vi "Select XNET Signals UI.vi"(8 "error in (no error)":errorcluster, 9 "XNET Cluster":refnum<k21>, 10 "XNET Database":refnum<k21>, 11 "Node Ptr":u64 format="%.0x") -> (0 "error out":errorcluster, 2 "Cancel Out":bool)   [LabVIEW 2019, in "Ghost Bus Addon System Explorer.lvlib"]
uses:
  Ghost Bus Addon System Explorer.lvlib
  <vilib>/Utility/cursorutil.llb/Set Cursor (Icon Pict).vi
panel:
  in  "Cancel":bool
  in  "Select":bool
  in  "Tree":string(tree)
  # "OUTPUTS"
  # "INPUTS"
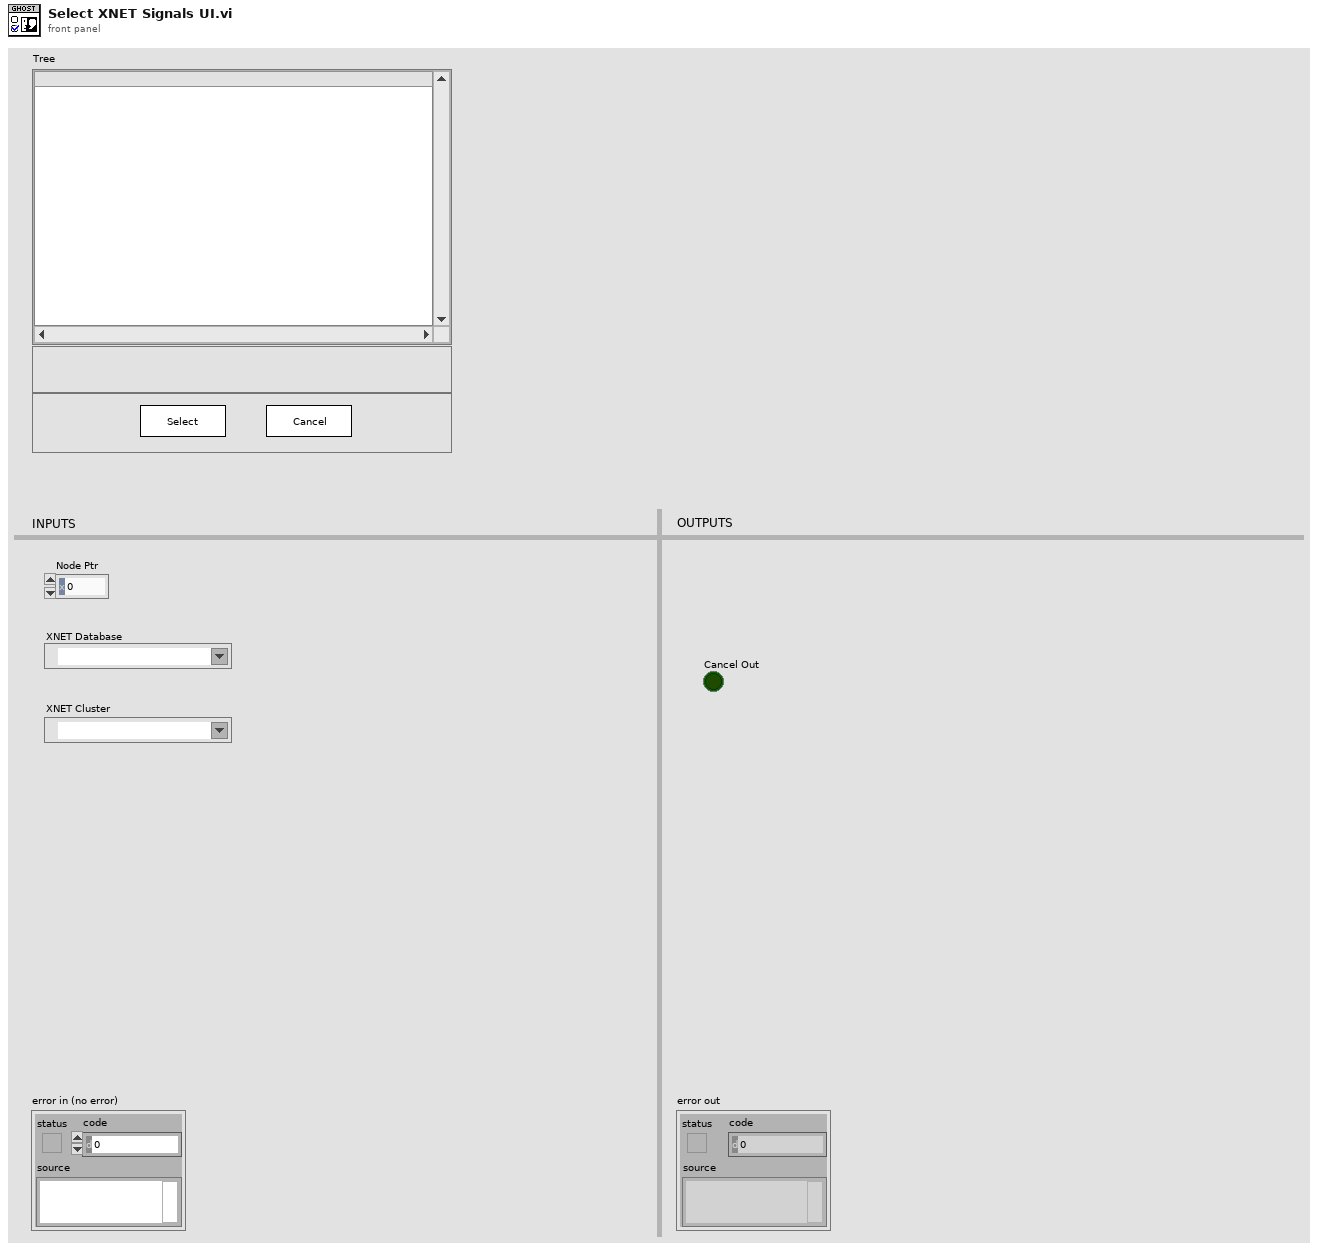
[diagram p1: front panel]
types:
  T1 = typedef "LVPoint32TypeDef.ctl" = cluster{"Horizontal":i32, "Vertical":i32}
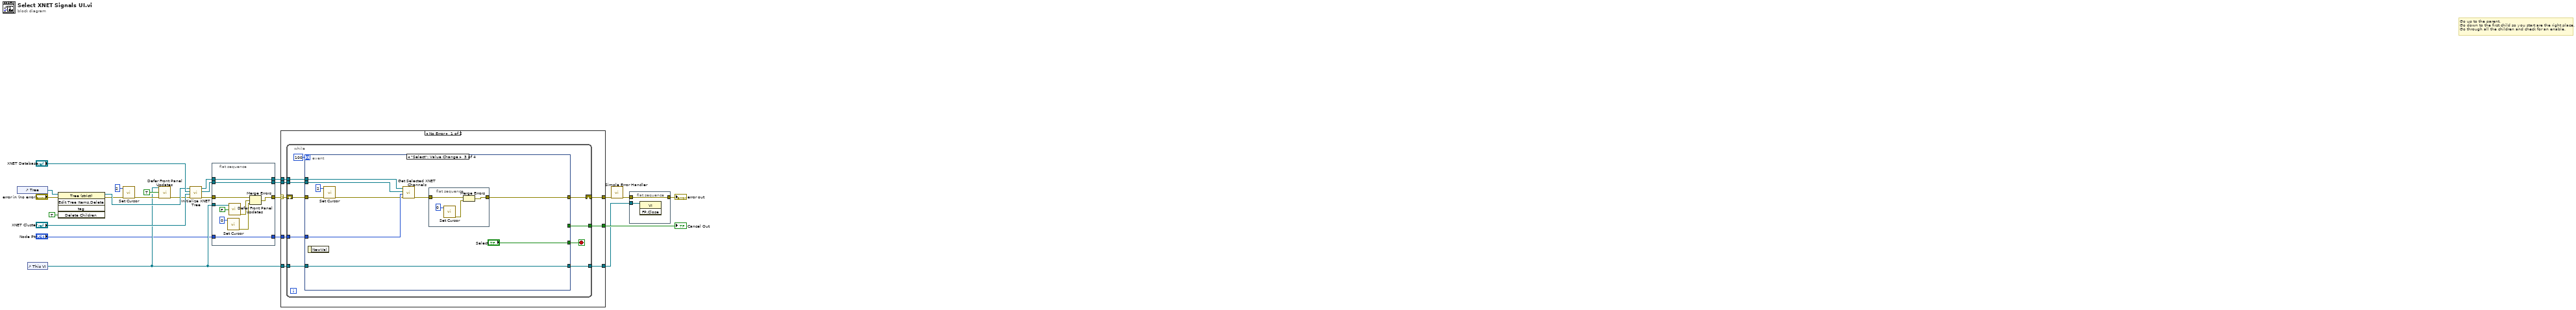
[diagram p0: block diagram]
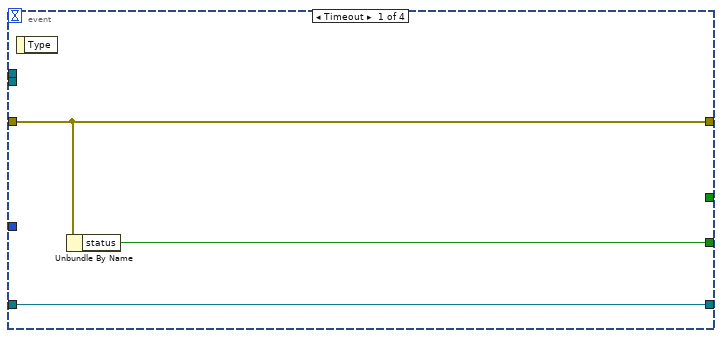
[diagram p2: hidden frame]
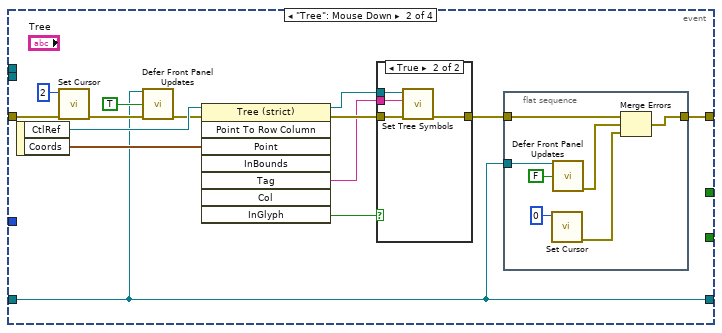
[diagram p3: hidden frame]
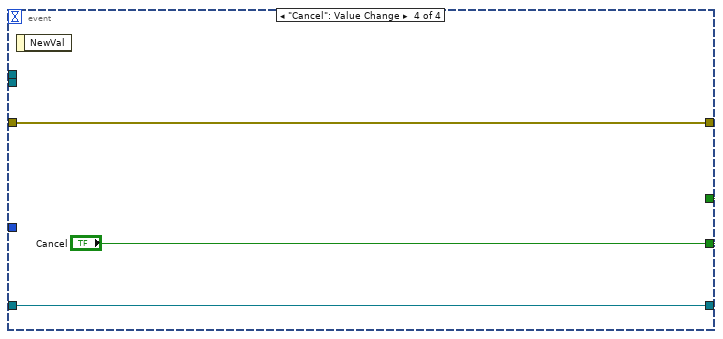
[diagram p5: hidden frame]
diagram:
  # "Go up to the parent.\nGo down to the first child so you start are the right place.\nGo through all the children and check for an enable."
  n1 = control-ref of="Tree"() -> (w13:refnum<vi>)
  n2 = control-ref of="This VI"() -> (w6:refnum<vi>)
  n3 = invoke on="Invoke Node" class="Tree (strict)" method="Edit Tree Items.Delete"(reference=w13, error in="error in (no error)", "Delete Children"=TRUE ("Delete Children?")) -> (reference out=w12:refnum<vi>, error out=w10:errorcluster)  [unwired: 2 in, 3 out]
  n4 = call-poly <vilib>:"Set Cursor.vi"("error in (no error)"=w10, "icon"=u16 2) -> ("error out"=w9:errorcluster)  [unwired: 8 in, 1 out]
  n5 = call "Defer Front Panel Updates.vi"("This VI"=w6, "Defer Panel Updates"=TRUE, "error in (no error)"=w9) -> ("error out"=w4:errorcluster)  [unwired: 12 in]
  n6 = call "Initialize XNET Tree.vi"("error in"=w4, "XNET Cluster"="XNET Cluster", "XNET Database"="XNET Database", "Tree"=w12) -> ("error out"=w3:errorcluster, "XNET Cluster Out"=w17:refnum<k21>, "Tree Out"=w1:refnum<vi>)  [unwired: 4 in, 1 out]
  n7 = flat-sequence {
    tunnel: [w34] -> w22
    tunnel: [w31] -> w21
    tunnel: [w29] -> w18
    tunnel: [w28] -> w7
    tunnel: w3 -> [w33]
    tunnel: w1 -> [w31]
    tunnel: w6 -> [w30]
    tunnel: w17 -> [w29]
    tunnel: "Node Ptr" -> [w28]
    frame #0 {
      n8 = call-poly <vilib>:"Set Cursor.vi"("icon"=u16 0) -> ("error out"=w26:errorcluster)  [unwired: 9 in, 1 out]
      n9 = call "Defer Front Panel Updates.vi"("This VI"=w30, "Defer Panel Updates"=FALSE) -> ("error out"=w32:errorcluster)  [unwired: 13 in]
      n10 = Merge Errors(w33, w32, w26) -> (w34:errorcluster)
    }
  }
  n11 = case shown="No Error" w22 {
    selector: w22 -> [w40 w101]
    tunnel: [w43 w101] -> w16
    tunnel: [w42 _] -> w25
    tunnel: w7 -> [w41 _]
    tunnel: w21 -> [w39 _]
    tunnel: w18 -> [w38 _]
    tunnel: w6 -> [w37 w100]
    tunnel: [w36 w100] -> w5
    frame No Error {
      n12 = while {
        shift-right: [w51] -> w43
        shift-left: w40 -> [w53]
        tunnel: w38 -> [w50]
        tunnel: [w49] -> w42
        tunnel: w41 -> [w48]
        tunnel: w39 -> [w47]
        tunnel: w37 -> [w45]
        tunnel: [w44] -> w36
        stop <- w52 stop-if-true
        n13 = event shown="[2] \"Select\": Value Change" {
          selector: _ -> [_ _ _ _]
          dyn-events: _ -> [_ _ _ _]
          timeout: 100 -> [_ _ _ _]
          tunnel: w53 -> [w56 w63 w87 w99]
          tunnel: [w55 _ "Select" "Cancel"] -> w52
          tunnel: [w56 w61 w86 w99] -> w51
          tunnel: w50 -> [_ _ w91 _]
          tunnel: [_ _ _ "Cancel"] -> w49
          tunnel: w48 -> [_ _ w90 _]
          tunnel: w47 -> [_ _ w89 _]
          tunnel: w45 -> [w54 w57 w84 w97]
          tunnel: [w54 w57 w84 w97] -> w44
          event Timeout {
            n14 = event-data() -> ()  [unwired: 1 in, 1 out]
            n15 = Unbundle By Name(w56) -> ("status"=w55:bool)
          }
          event "Tree": Mouse Down {
            n16 = event-data() -> ("CtlRef"=w69:refnum<vi>, "Coords"=w70:T1)  [unwired: 1 in]
            n17 = call-poly <vilib>:"Set Cursor.vi"("error in (no error)"=w63, "icon"=u16 2) -> ("error out"=w59:errorcluster)  [unwired: 8 in, 1 out]
            n18 = call "Defer Front Panel Updates.vi"("This VI"=w57, "Defer Panel Updates"=TRUE, "error in (no error)"=w59) -> ("error out"=w58:errorcluster)  [unwired: 12 in]
            n19 = invoke on="Invoke Node" class="Tree (strict)" method="Point To Row Column"(reference=w69, error in=w58, "Point"=w70) -> (reference out=w67:refnum<vi>, error out=w68:errorcluster, "Tag"=w66:string, "InGlyph"=w65:bool)  [unwired: 5 in, 4 out]
            n20 = case shown="True" w65 {
              tunnel: w68 -> [w78 w82]
              tunnel: w67 -> [_ w81]
              tunnel: w66 -> [_ w80]
              tunnel: [w78 w79] -> w62
              frame False {
              }
              frame True {
                n21 = call "Set Tree Symbols.vi"("error in"=w82, "Tag"=w80, "CtlRef"=w81) -> ("error out"=w79:errorcluster)  [unwired: 8 in]
              }
            }
            n22 = flat-sequence {
              tunnel: [w74] -> w61
              tunnel: w62 -> [w75]
              tunnel: w57 -> [w71]
              frame #0 {
                n23 = call-poly <vilib>:"Set Cursor.vi"("icon"=u16 0) -> ("error out"=w76:errorcluster)  [unwired: 9 in, 1 out]
                n24 = call "Defer Front Panel Updates.vi"("This VI"=w71, "Defer Panel Updates"=FALSE) -> ("error out"=w72:errorcluster)  [unwired: 13 in]
                n25 = Merge Errors(w75, w72, w76) -> (w74:errorcluster)
              }
            }
          }
          event "Select": Value Change {
            n26 = event-data() -> ()  [unwired: 1 in, 1 out]
            n27 = call-poly <vilib>:"Set Cursor.vi"("error in (no error)"=w87, "icon"=u16 2) -> ("error out"=w83:errorcluster)  [unwired: 8 in, 1 out]
            n28 = call "Get Selected XNET Channels.vi"("error in (no error)"=w83, "Node Ptr"=w90, "XNET Cluster"=w91, "Tree In"=w89) -> ("error out"=w85:errorcluster)  [unwired: 6 in, 1 out]
            n29 = flat-sequence {
              tunnel: [w93] -> w86
              tunnel: w85 -> [w94]
              frame #0 {
                n30 = call-poly <vilib>:"Set Cursor.vi"("icon"=u16 0) -> ("error out"=w95:errorcluster)  [unwired: 9 in, 1 out]
                n31 = Merge Errors(w94, w95) -> (w93:errorcluster)
              }
            }
          }
          event "Cancel": Value Change {
            n32 = event-data() -> ()  [unwired: 1 in, 1 out]
          }
        }
      }
    }
    frame Error {
    }
  }
  "Cancel Out" <- w25
  n33 = call <vilib>:"Simple Error Handler.vi"("error in (no error)"=w16) -> ("error out"=w15:errorcluster)  [unwired: 4 in, 4 out]
  n34 = flat-sequence {
    tunnel: [w103] -> w23
    tunnel: w15 -> [w103]
    tunnel: w5 -> [w102]
    frame #0 {
      n35 = invoke class="VI" method="FP.Close"(reference=w102) -> ()  [unwired: 2 in, 3 out]
    }
  }
  "error out" <- w23
